vi "Post-Register.vi"(8 "error in (no error)":errorcluster, 11 "Configuration Editor in":refnum<class "Configuration Editor.lvclass">) -> (0 "error out":errorcluster, 3 "Configuration Editor out":refnum<class "Configuration Editor.lvclass">)   [LabVIEW 2023, in "Configuration Editor.lvlib" / "Configuration Editor.lvclass"]
doc: "<b>Post Register</b>\nThis routine is implemented in <b>Post Launch Initialize</b> after the actor has registered for events.\n\nIt's intended to provide a means of performing actions immediately before the actor state engine is entered."
uses:
  Library/Configuration Editor.lvclass
  Library/Configuration Editor.lvclass/Configuration Editor.ctl
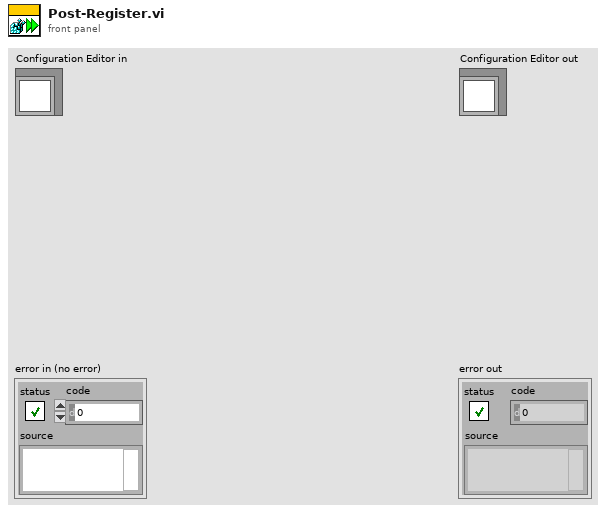
[diagram p1: front panel]
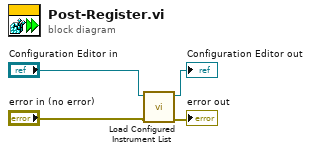
[diagram p0: block diagram]
diagram:
  n1 = call "Load Configured Instrument List.vi"("error in (no error)"="error in (no error)", "Configuration Editor in"="Configuration Editor in") -> ("error out"=→"error out":errorcluster, "Configuration Editor out"=→"Configuration Editor out":refnum<class "Configuration Editor.lvclass">)  [unwired: 8 in]
